vi "DGHD5331_3R.vi"() -> ()   [LabVIEW 2014]
uses:
  <vilib>/Instr/_visa.llb/VISA Configure Serial Port (Instr).vi
  <vilib>/Utility/file.llb/Write To Spreadsheet File (string).vi
panel:
  out "Run time":string
  in  "Unit 2":string
  in  "Additional 2":sgl min=-1000 max=1000 step=0.1
  in  "Unit":string
  in  "Additional 1":sgl min=-1000 max=1000 step=0.1
  out "Time/Date":string
  out "No of samples":i32
  out "Raw Data Read":string
  out "Bytes Read":u32
  in  "Comm Port":refnum<visa-resource-name>
  in  "Sample rate (s)":u8=100
  out "Waveform Chart":dynamicdata(graph)
  in  "stop":bool
  # "Optional \nAdditional numeric info \n(Voltage, Curent, Power)\n\nWill be logged to file"
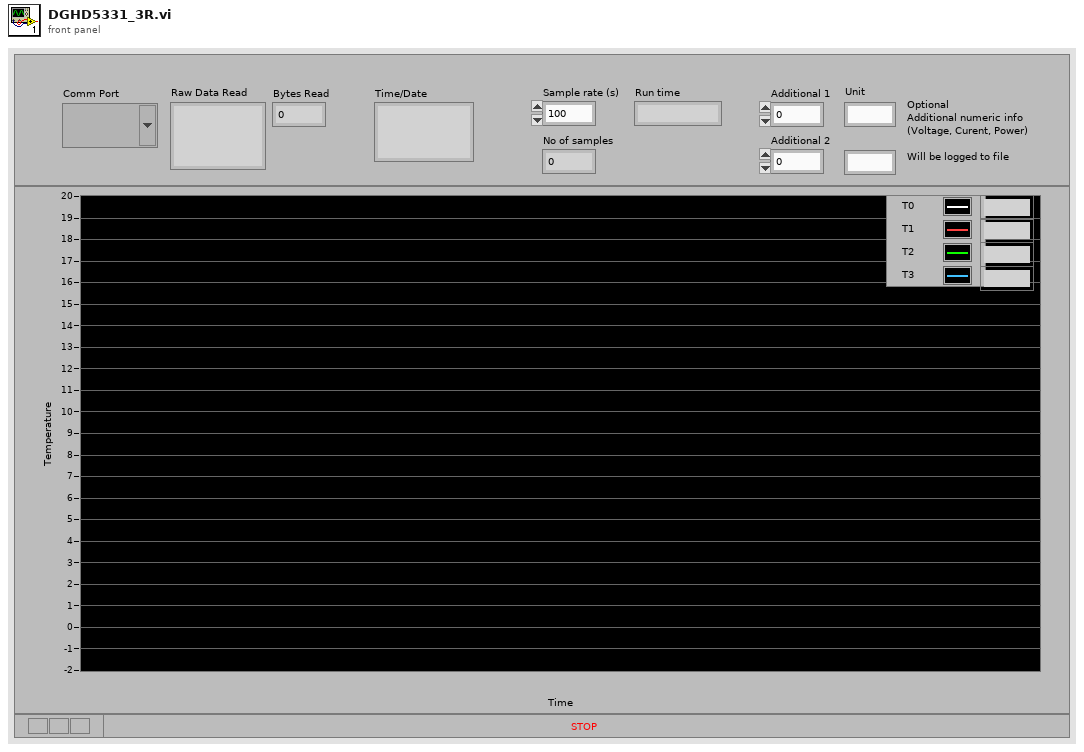
[diagram p1: front panel]
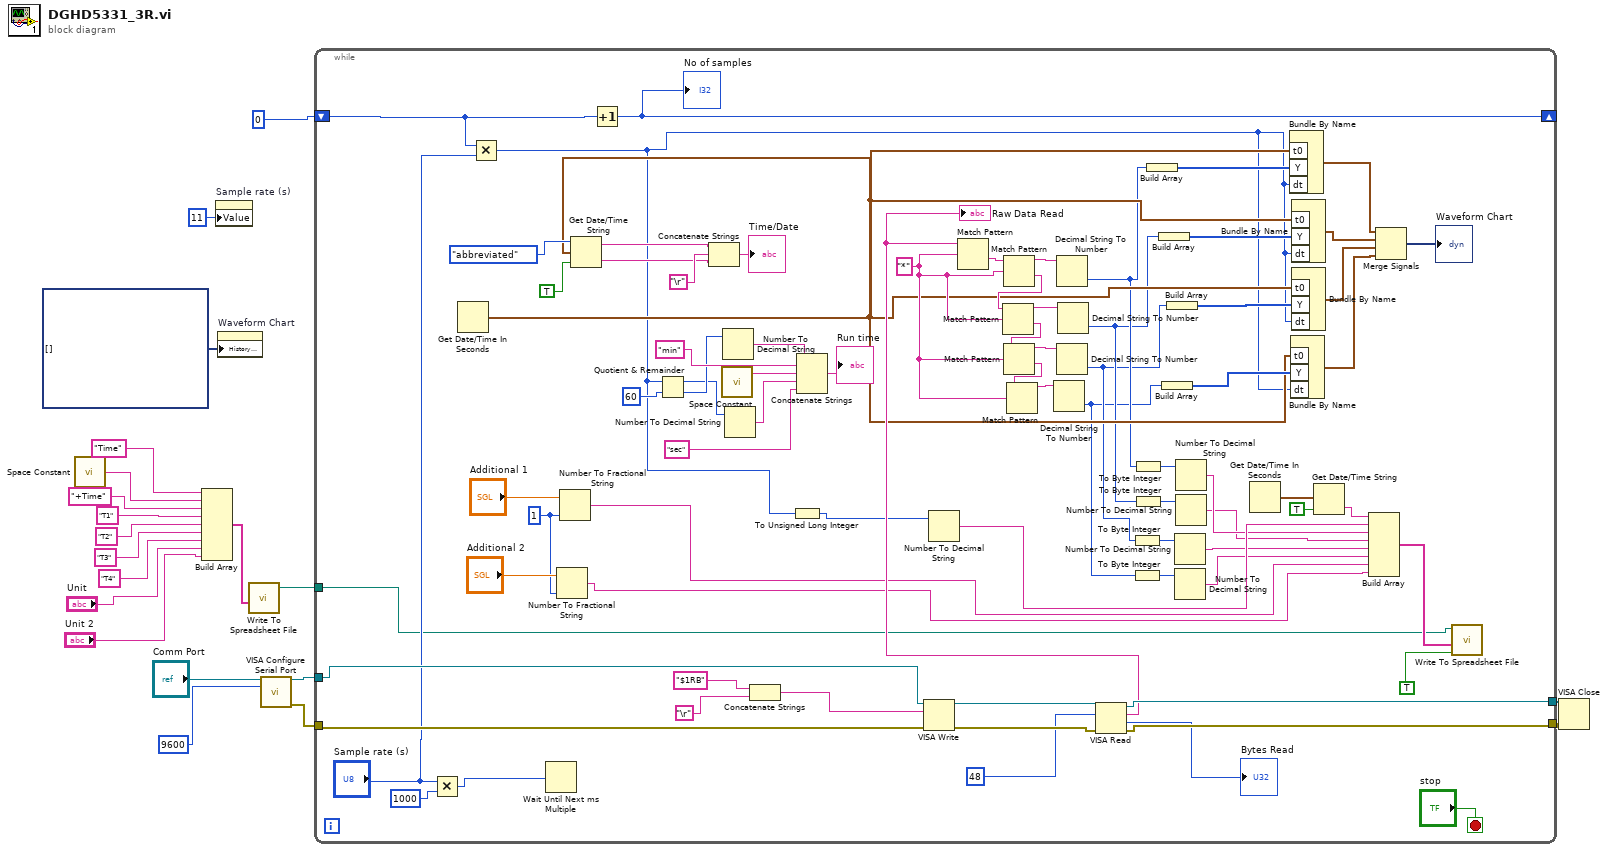
[diagram p0: block diagram]
diagram:
  n1 = call <vilib>:"Space Constant.vi"() -> ("String"=w5:string)
  n2 = Build Array("Time" ("element"), w5, "+Time", "T1", "T2", "T3", "T4", "Unit", "Unit 2") -> (w8:string[])
  n3 = property on="Sample rate (s)" class="DigNum (strict)"("Value"=u8 11 ("Sample rate (s)")) -> ()  [unwired: 2 in, 2 out]
  n4 = property on="Waveform Chart" class="WFChart (strict)"("History Data"=dynamicdata[] []) -> ()  [unwired: 2 in, 2 out]
  n5 = call-poly <vilib>:"Write To Spreadsheet File.vi"("1D data"=w8) -> ("new file path (Not A Path if cancelled)"=w4:path)  [unwired: 7 in]
  n6 = call-poly "VISA Configure Serial Port"("VISA resource name"="Comm Port", "baud rate (9600)"=9600) -> ("VISA resource name out"=w19:refnum<visa-resource-name>, "error out"=w17:errorcluster)  [unwired: 12 in]
  n7 = while {
    tunnel: w19 -> [w97]
    tunnel: w17 -> [w96]
    tunnel: [w93] -> w16
    tunnel: [w92] -> w15
    shift-right: [w77] -> _
    shift-left: 0 -> [w60]
    tunnel: w4 -> [w31]
    stop <- "stop" stop-if-true
    w34 = i16 1 ("precision (6)")
    w81 = "*"
    n8 = Multiply(x="Sample rate (s)", y=1000) -> (x*y=w38:i32)
    n9 = Get Date/Time In Seconds() -> (seconds since 1Jan1904=w64:timestamp)
    n10 = Multiply(x=w60, y="Sample rate (s)") -> (x*y=w29:i32)
    n11 = Wait Until Next ms Multiple(millisecond multiple=w38) -> ()  [unwired: 1 out]
    n12 = Number To Fractional String(number="Additional 2", precision (6)=w34) -> (F-format string=w32:string)  [unwired: 2 in]
    n13 = Number To Fractional String(number="Additional 1", precision (6)=w34) -> (F-format string=w33:string)  [unwired: 2 in]
    n14 = Get Date/Time String(date format (0)=enum16{"short", "long", "abbreviated"}."abbreviated", seconds (now)=w64, want seconds? (F)=TRUE) -> (date string=w59:string, time string=w58:string)
    n15 = Increment(x=w60) -> (x+1=w77:i32)
    "No of samples" <- w77
    n16 = Quotient & Remainder(x=w29, y=60) -> (x-y*floor(x/y)=w24:i32, floor(x/y)=w25:i32)
    n17 = Concatenate Strings(w59, "\r", w58) -> (→"Time/Date":string)
    n18 = call <vilib>:"Space Constant.vi"() -> ("String"=w23:string)
    n19 = Number To Decimal String(number=w25) -> (decimal integer string=w27:string)  [unwired: 1 in]
    n20 = Number To Decimal String(number=w24) -> (decimal integer string=w22:string)  [unwired: 1 in]
    n21 = Concatenate Strings("$1RB", "\r") -> (w88:string)
    n22 = To Unsigned Long Integer(number=w29) -> (unsigned 32bit integer=w54:u32)
    n23 = Concatenate Strings(w27, "min", w23, w22, "sec") -> (→"Run time":string)
    n24 = VISA Write(VISA resource name=w97, write buffer=w88, error in (no error)=w96) -> (VISA resource name out=w95:refnum<visa-resource-name>, error out=w94:errorcluster)  [unwired: 1 out]
    n25 = Number To Decimal String(number=w54) -> (decimal integer string=w53:string)  [unwired: 1 in]
    n26 = VISA Read(VISA resource name=w95, byte count=u32 48 ("Bytes Read"), error in (no error)=w94) -> (VISA resource name out=w93:refnum<visa-resource-name>, read buffer=w76:string, return count=→"Bytes Read":u32, error out=w92:errorcluster)
    "Raw Data Read" <- w76
    n27 = Match Pattern(string=w76, regular expression=w81) -> (after substring=w87:string)  [unwired: 1 in, 3 out]
    n28 = Match Pattern(string=w87, regular expression=w81) -> (before substring=w86:string, after substring=w84:string)  [unwired: 1 in, 2 out]
    n29 = Match Pattern(string=w84, regular expression=w81) -> (before substring=w85:string, after substring=w80:string)  [unwired: 1 in, 2 out]
    n30 = Match Pattern(string=w80, regular expression=w81) -> (before substring=w83:string, after substring=w79:string)  [unwired: 1 in, 2 out]
    n31 = Match Pattern(string=w79, regular expression=w81) -> (before substring=w82:string)  [unwired: 1 in, 3 out]
    n32 = Decimal String To Number(string=w82) -> (number=w45:i32)  [unwired: 2 in, 1 out]
    n33 = Decimal String To Number(string=w86) -> (number=w48:i32)  [unwired: 2 in, 1 out]
    n34 = Decimal String To Number(string=w83) -> (number=w46:i32)  [unwired: 2 in, 1 out]
    n35 = Decimal String To Number(string=w85) -> (number=w47:i32)  [unwired: 2 in, 1 out]
    n36 = To Byte Integer(number=w46) -> (8bit integer=w50:i8)
    n37 = To Byte Integer(number=w45) -> (8bit integer=w49:i8)
    n38 = To Byte Integer(number=w48) -> (8bit integer=w52:i8)
    n39 = To Byte Integer(number=w47) -> (8bit integer=w51:i8)
    n40 = Build Array(w48) -> (w72:i32[])
    n41 = Build Array(w47) -> (w71:i32[])
    n42 = Build Array(w45) -> (w69:i32[])
    n43 = Build Array(w46) -> (w70:i32[])
    n44 = Number To Decimal String(number=w50) -> (decimal integer string=w42:string)  [unwired: 1 in]
    n45 = Number To Decimal String(number=w49) -> (decimal integer string=w41:string)  [unwired: 1 in]
    n46 = Number To Decimal String(number=w52) -> (decimal integer string=w44:string)  [unwired: 1 in]
    n47 = Number To Decimal String(number=w51) -> (decimal integer string=w43:string)  [unwired: 1 in]
    n48 = Get Date/Time In Seconds() -> (seconds since 1Jan1904=w56:timestamp)
    n49 = Bundle By Name("t0"=w64, "Y"=w72, "dt"=w29) -> (w63:waveform(i32))  [unwired: 1 in]
    n50 = Bundle By Name("t0"=w64, "Y"=w69, "dt"=w29) -> (w65:waveform(i32))  [unwired: 1 in]
    n51 = Bundle By Name("t0"=w64, "Y"=w71, "dt"=w29) -> (w62:waveform(i32))  [unwired: 1 in]
    n52 = Bundle By Name("t0"=w64, "Y"=w70, "dt"=w29) -> (w61:waveform(i32))  [unwired: 1 in]
    n53 = Get Date/Time String(seconds (now)=w56, want seconds? (F)=TRUE) -> (time string=w55:string)  [unwired: 1 in, 1 out]
    n54 = Build Array(w55, w53, w44, w43, w42, w41, w33, w32) -> (w57:string[])
    n55 = Merge Signals(w63, w62, w61, w65) -> (→"Waveform Chart":dynamicdata)
    n56 = call-poly <vilib>:"Write To Spreadsheet File.vi"("append to file? (new file:F)"=TRUE, "1D data"=w57, "file path (dialog if empty)"=w31) -> ()  [unwired: 5 in, 1 out]
  }
  n57 = VISA Close(VISA resource name=w16, error in (no error)=w15) -> ()  [unwired: 1 out]
